vi "_PC_Pub_GenerateErrorCode.vi"(2 "String to Prepend to source (\"\")":string, 3 "error in":errorcluster, 4 "status":bool, 5 "Ring":i32(ring) items=["No error", "Argument error", "Memory is full", "Out of zone", "End of file", "File already open", "Generic file I/O error", "File not found", "File permission error", "Disk is full", "Duplicate path", "Too many files open", "System feature not enabled", "Resource file not found", "Cannot add resource", "Resource not found", "Image not found", "Image memory error", "Pen does not exist", "Config type invalid", "Config token not found", "Config parse error", "Config memory error", "Bad external code format", "Bad external code offset", "External code not present", "Null window", "Destroy window error", "Null menu", "Print aborted", "Bad print record", "Print driver error", "Windows error during printing", "Memory error during printing", "Print dialog error", "Generic print error", "Invalid device refnum", "Device not found", "Device parameter error", "Device unit error", "Cannot open device", "Device call aborted", "Generic error", "Cancelled by user", "Object ID too low", "Object ID too high", "Object not in heap", "Unknown heap", "Unknown object (invalid DefProc)", "Unknown object (DefProc not in table)", "Message out of range", "Invalid (null) method", "Unknown message", "Manager call not supported", "Bad address", "Network operation in progress", "Network operation timed out", "Connection is busy", "Network attribute not supported", "Network error", "Address in use", "System out of memory", "Connection aborted", "Connection refused", "Not connected", "Already connected", "Connection closed", "Initialization error (interapplication manager)", "Bad occurrence", "Wait on unbound occurrence handler", "Occurrence queue overflow", "Datalog type conflict", "Unused", "Unrecognized type (interapplication manager)", "Memory corrupt", "Failed to make temporary DLL", "Old CIN version", "Drag socket not found", "Failed to load drop-object", "Failed to register OLE object", "Failed to release OLE object", "Format specifier type mismatch", "Unknown format specifier", "Too few format specifiers", "Too many format specifiers", "Scan failed", "Newer CIN version", "Error converting to variant", "Runtime menu error", "Password tampered", "Variant attribute not found", "Incompatible variant data type", "Event data is not available", "Event Store is not present", "Occurrence is not found", "Event Queue is not created", "Event info is not available", "Refnum passed is NULL", "Error retrieving Class GUID", "Error retrieving CoClass GUID", "Error retrieving TypeLib GUID.", "Bad built application magic bytes.", "Specific driver is different from the specific driver associated with the Logical Name.", "There is no session opened to the class driver.", "Max Error", "MAX - Error with config objects", "MAX - Error loading configuration", "MAX - Group not supported", "Times Out"]) -> (0 "error out":errorcluster)   [LabVIEW 2018]
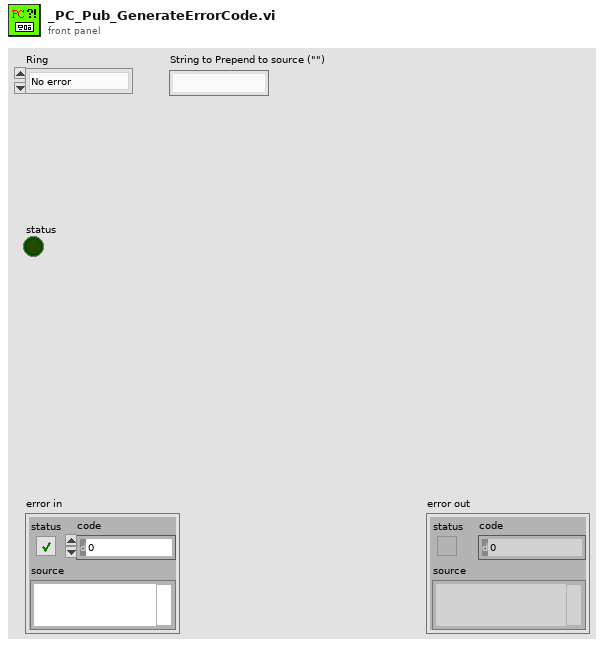
[diagram p1: front panel]
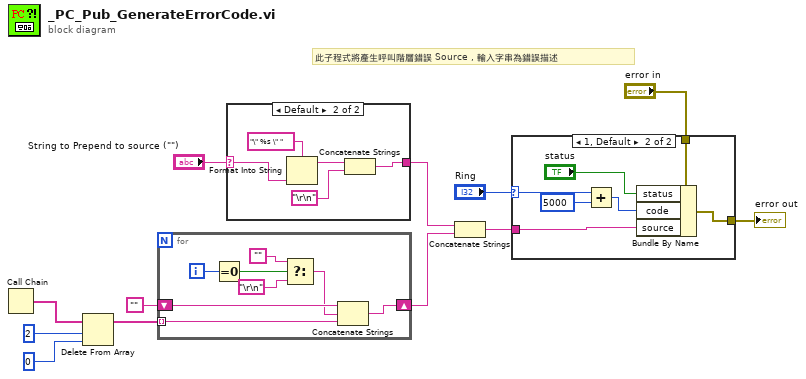
[diagram p0: block diagram]
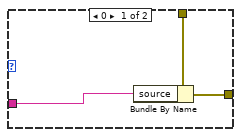
[diagram p2: hidden frame]
diagram:
  # "此子程式將產生呼叫階層錯誤 Source , 輸入字串為錯誤描述"
  n1 = Call Chain() -> (call chain=w12:string[])
  n2 = Delete From Array(array=w12, length=2 ("Length"), index=0 ("Index")) -> (array with subset deleted=w8:string[])  [unwired: 1 out]
  n3 = for {
    tunnel: w8 -> [w14] mode=indexing
    shift-right: [w19] -> w5
    shift-left: "" -> [w20]
    i -> [w18]
    n4 = Equal To 0?(x=w18) -> (x = 0?=w17:bool)
    n5 = Select(t="", s=w17, f="\r\n") -> (s? t:f=w13:string)
    n6 = Concatenate Strings(w20, w13, w14) -> (w19:string)
  }
  n7 = case shown="Default" "String to Prepend to source (\"\")" {
    selector: "String to Prepend to source (\"\")" -> [w21 w26]
    tunnel: [w21 w22] -> w6
    frame "" {
    }
    frame Default {
      n8 = Format Into String(format string="\" %s \" " ("Format String"), w26) -> (resulting string=w24:string)  [unwired: 2 in, 1 out]
      n9 = Concatenate Strings(w24, "\r\n") -> (w22:string)
    }
  }
  n10 = Concatenate Strings(w6, w5) -> (w9:string)
  n11 = case shown="1, Default" "Ring" {
    selector: "Ring" -> [_ w33]
    tunnel: w9 -> [w29 w36]
    tunnel: [w28 w35] -> w4
    tunnel: "error in" -> [w27 w34]
    frame 0 {
      n12 = Bundle By Name(cluster=w27, "source"=w29) -> (w28:errorcluster)
    }
    frame 1, Default {
      n13 = Add(x=w33, y=5000) -> (x+y=w31:i32)
      n14 = Bundle By Name(cluster=w34, "status"="status", "code"=w31, "source"=w36) -> (w35:errorcluster)
    }
  }
  "error out" <- w4
